vi "LOC subReadWriteVIStringINIKeys(Slide).vi"(4 "Mode":enum16{"Read", "Write"}(ring), 5 "Section":string, 6 "error in (no error)":errorcluster, 8 "ConfigFileRefnum":T1, 9 "ControlRefnum":refnum<vi>) -> (0 "error out":errorcluster)   [LabVIEW 2020, in "Localization_Tools.lvlib"]
uses:
  Localization_Tools.lvlib
  <vilib>/Utility/config.llb/Config Data RefNum.ctl
  <vilib>/Utility/config.llb/NI_LVConfig.lvlib
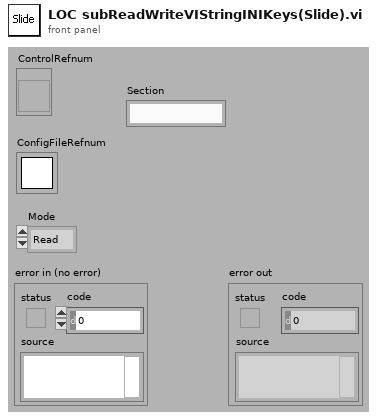
[diagram p1: front panel]
types:
  T1 = typedef "NI_LVConfig.lvlib/Config Data RefNum.ctl" = refnum<k1>
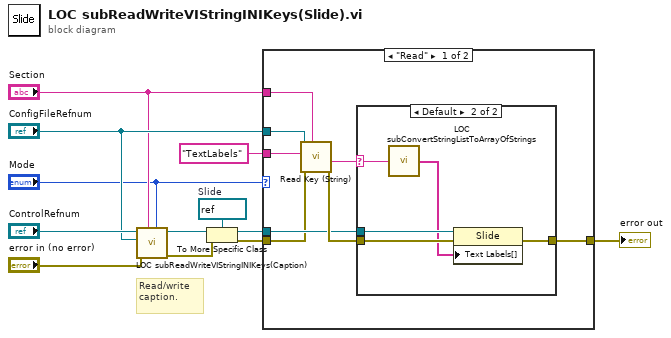
[diagram p0: block diagram]
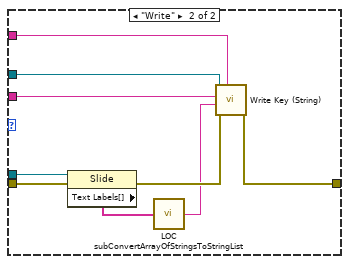
[diagram p3: hidden frame]
diagram:
  w5 = refnum<vi> refnum  # Slide
  # "Read/write\ncaption."
  n1 = call "LOC subReadWriteVIStringINIKeys(Caption).vi"("Mode"="Mode", "Section"="Section", "error in (no error)"="error in (no error)", "ConfigFileRefnum"="ConfigFileRefnum", "ControlRefnum"="ControlRefnum") -> ("error out"=w2:errorcluster, "dup ControlRefnum"=w4:refnum<vi>)  [unwired: 3 in]
  n2 = To More Specific Class(target class=w5, reference=w4, error in=w2) -> (specific class reference=w3:refnum<vi>, error out=w1:errorcluster)
  n3 = case shown="\"Read\"" "Mode" {
    tunnel: w3 -> [w14 w28]
    tunnel: w1 -> [w13 w27]
    tunnel: "ConfigFileRefnum" -> [w20 w35]
    tunnel: "Section" -> [w19 w33]
    tunnel: "TextLabels" ("key") -> [w18 w34]
    tunnel: [w16 w31] -> w6
    frame "Read" {
      n4 = call <vilib>:"Read Key (String).vi"("section"=w19, "error in (no error)"=w13, "key"=w18, "refnum"=w20) -> ("error out"=w17:errorcluster, "value"=w15:string)  [unwired: 4 in, 2 out]
      n5 = case shown="Default" w15 {
        selector: w15 -> [_ w22]
        tunnel: w14 -> [_ w26]
        tunnel: w17 -> [w21 w25]
        tunnel: [w21 w24] -> w16
        frame "" {
        }
        frame Default {
          n6 = call "LOC subConvertStringListToArrayOfStrings.vi"("InputString"=w22) -> ("OutputArray"=w23:string[])
          n7 = property class="Slide"(reference=w26, error in=w25, "Text Labels[]"=w23) -> (error out=w24:errorcluster)  [unwired: 1 out]
        }
      }
    }
    frame "Write" {
      n8 = property class="Slide"(reference=w28, error in=w27) -> (error out=w32:errorcluster, "Text Labels[]"=w30:string[])  [unwired: 1 out]
      n9 = call "LOC subConvertArrayOfStringsToStringList.vi"("InputArray"=w30) -> ("OutputString"=w29:string)
      n10 = call <vilib>:"Write Key (String).vi"("section"=w33, "error in (no error)"=w32, "value"=w29, "key"=w34, "refnum"=w35) -> ("error out"=w31:errorcluster)  [unwired: 4 in, 2 out]
    }
  }
  "error out" <- w6
